vi "round2mV (SubVI).vi"(11 "Numeric in":sgl) -> (3 "Numeric out":dbl)   [LabVIEW 2014]
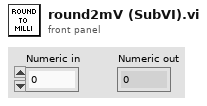
[diagram p1: front panel]
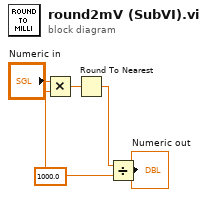
[diagram p0: block diagram]
diagram:
  w3 = 1000.0 ("y")
  n1 = Multiply(x="Numeric in", y=w3) -> (x*y=w1:dbl)
  n2 = Round To Nearest(number=w1) -> (nearest integer value=w2:dbl)
  n3 = Divide(x=w2, y=w3) -> (x/y=→"Numeric out":dbl)
